vi "Add RF Connection.vi"(6 "Overwrite (On)":bool=TRUE, 7 "Connector (\"Connector1\")":string="Connector1", 8 "error in (no error)":errorcluster, 9 "Antenna (\"RRH\")":string="RRH", 10 "RF Connection (\"LTE Main\")":string="LTE Main", 11 "VISA resource name":refnum<visa-resource-name>) -> (0 "error out":errorcluster, 3 "VISA resource name out":refnum<visa-resource-name>)   [LabVIEW 2020, in "Rohde&Schwarz CMXP Base.lvlib"]
doc: "Creates a signal path for a selected connector and assigns a name to the path.\n\nAssign a unique name to each named object within the test environment. Assigning an already used name can be rejected with an error message, even if the other object has not the same type as the new object.\n\nAttribute:\n-\n\nRemote-control command:\nCREate:TENVironment:SPATh"
uses:
  <instrlib>/Rohde&Schwarz CMXP Base/Rohde&Schwarz CMXP Base.lvlib
  <instrlib>/Rohde&Schwarz CMXP Base/Private/rsidr_core.llb/rsidr_core.lvlib
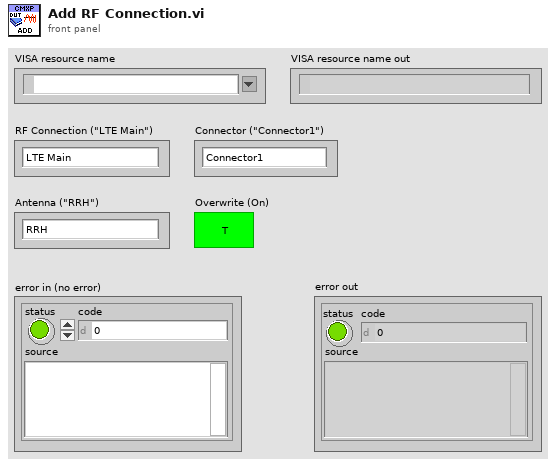
[diagram p1: front panel]
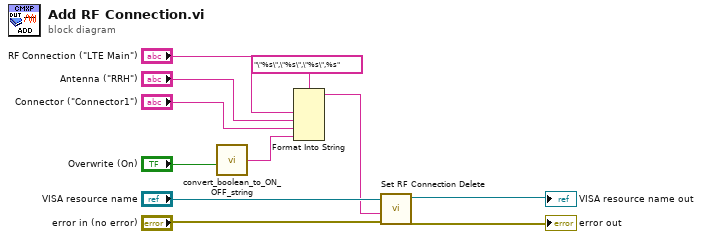
[diagram p0: block diagram]
diagram:
  n1 = call <instrlib>:"convert_boolean_to_ON_OFF_string.vi"("boolean value in"="Overwrite (On)") -> ("string value out"=w3:string)  [unwired: 4 in]
  n2 = Format Into String(format string="\"%s\",\"%s\",\"%s\",%s", "RF Connection (\"LTE Main\")", "Antenna (\"RRH\")", "Connector (\"Connector1\")", w3) -> (resulting string=w1:string)  [unwired: 2 in, 1 out]
  n3 = call "Set RF Connection Delete"("error in (no error)"="error in (no error)", "RF Connection Delete ()"=w1, "instrument handle"="VISA resource name") -> ("error out"=→"error out":errorcluster, "instrument handle out"=→"VISA resource name out":refnum<visa-resource-name>)  [unwired: 7 in]
